vi "SplineParam_StackPop.vi"(11 "InputStack":T1) -> (1 "outputStack":T1, 2 "T1":dbl, 3 "T0":dbl)   [LabVIEW 2019, in "Trajectory_Library.lvlib"]
doc: "Internal routine used by SplineParam_Spline_T0_T1. This routine \"pops\", the item from the top of the stack and decrements the items on the stack.\n\nParameters:\n - InputStack - Stack data structure\n\nReturns:\n - OutputStack - Updated Stack data structure\n - T0\n - T1"
uses:
  Trajectory_Library.lvlib
  PARAM_STACK.ctl
  PARAM_STACK_ITEM.ctl
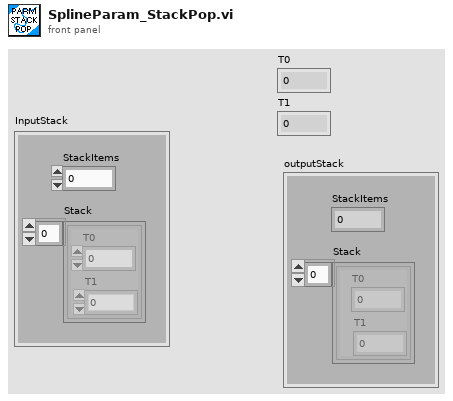
[diagram p1: front panel]
types:
  T1 = typedef "Trajectory_Library.lvlib/PARAM_STACK.ctl" = cluster{"StackItems":i32, "Stack":T2[]}
  T2 = typedef "Trajectory_Library.lvlib/PARAM_STACK_ITEM.ctl" = cluster{"T0":dbl, "T1":dbl}
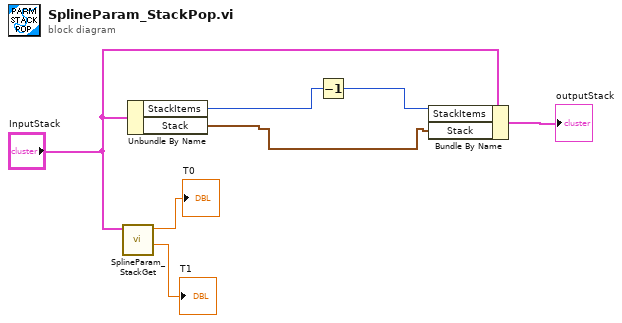
[diagram p0: block diagram]
diagram:
  n1 = call "SplineParam_StackGet.vi"("InputStack"="InputStack") -> ("T1"=→"T1":dbl, "T0"=→"T0":dbl)  [unwired: 9 in]
  n2 = Unbundle By Name("InputStack") -> ("StackItems"=w3:i32, "Stack"=w4:T2[])
  n3 = Decrement(x=w3) -> (x-1=w2:i32)
  n4 = Bundle By Name(cluster="InputStack", "StackItems"=w2, "Stack"=w4) -> (→"outputStack":T1)
